vi "Panel.vi"(11 "MultiPlotPanel in":refnum<class "MultiPlotPanel.lvclass">) -> ()   [LabVIEW 2021, in "MultiStokePlot.lvlib" / "MultiPlotPanel.lvclass"]
uses:
  MultiPlotPanel.lvclass
  C:/Program Files/National Instruments/LabVIEW 2021/vi.lib/IlluminatedG/IG OOPanel/OOPanel/Panel/Panel.lvclass
  SubVIs/Window Position and plot number.ctl
  SubVIs/Window Position.ctl
  SubVIs/Loop Data.ctl
  <vilib>/IlluminatedG/IG OOPanel/OOPanel/Manager/Manager.lvclass
  SubVIs/Panel Map.ctl
  SubVIs/Panel Map Data.ctl
  <userlib>/bjustice/RocketPlot/Classes/RocketPlotPanel/RocketPlotPanel.lvclass
  <vilib>/IlluminatedG/IG OOPanel/OOPanel/Panel/Panel Events.ctl
  <vilib>/IlluminatedG/IG OOPanel/OOPanel/Panel/Visbility Event Data.ctl
  <vilib>/IlluminatedG/IG OOPanel/OOPanel/Visibility State.ctl
  <vilib>/IlluminatedG/IG OOPanel/OOPanel/Close Reason.ctl
  <vilib>/Utility/miscctls.llb/LVPointTypeDef.ctl
  <userlib>/bjustice/RocketPlot/Classes/RocketPlotHandle/SubVIs/callback data.ctl
  <userlib>/bjustice/RocketPlot/Classes/RocketPlotHandle/SubVIs/callback type.ctl
  MultiPlotPanel.lvclass/MultiPlotPanel.ctl
  <userlib>/bjustice/RocketPlot/Classes/RocketPlotHandle/SubVIs/callback maximize data.ctl
  <vilib>/IlluminatedG/IG OOPanel/OOPanel/Panel/Panel.lvclass
  <userlib>/bjustice/RocketPlot/Classes/RocketPlotHandle/RocketPlotHandle.lvclass
  <vilib>/IlluminatedG/IG OOPanel/OOPanel/OOPanel.lvlib
panel:
  in  "Selection":T1[](array[typedef]) {"Plot Bounds (%)"."Bottom (%)" format="%.2f"; "Plot Bounds (%)"."Top (%)" format="%.2f"; "Plot Bounds (%)"."Right (%)" format="%.2f"; "Plot Bounds (%)"."Left (%)" format="%.2f"}
  in  "Select Layout (spoof)":bool
  in  "Select Layout":bool
  in  "Save Layout (spoof)":bool
  in  "Save Layout":bool
  in  "Load Layout (spoof)":bool
  in  "Load Layout":bool
  in  "Time to Plot":dbl=1800.0 format="%<%H:%M:%S>t"
  in  "Apply Time to Plot":bool
  out "Filename":string
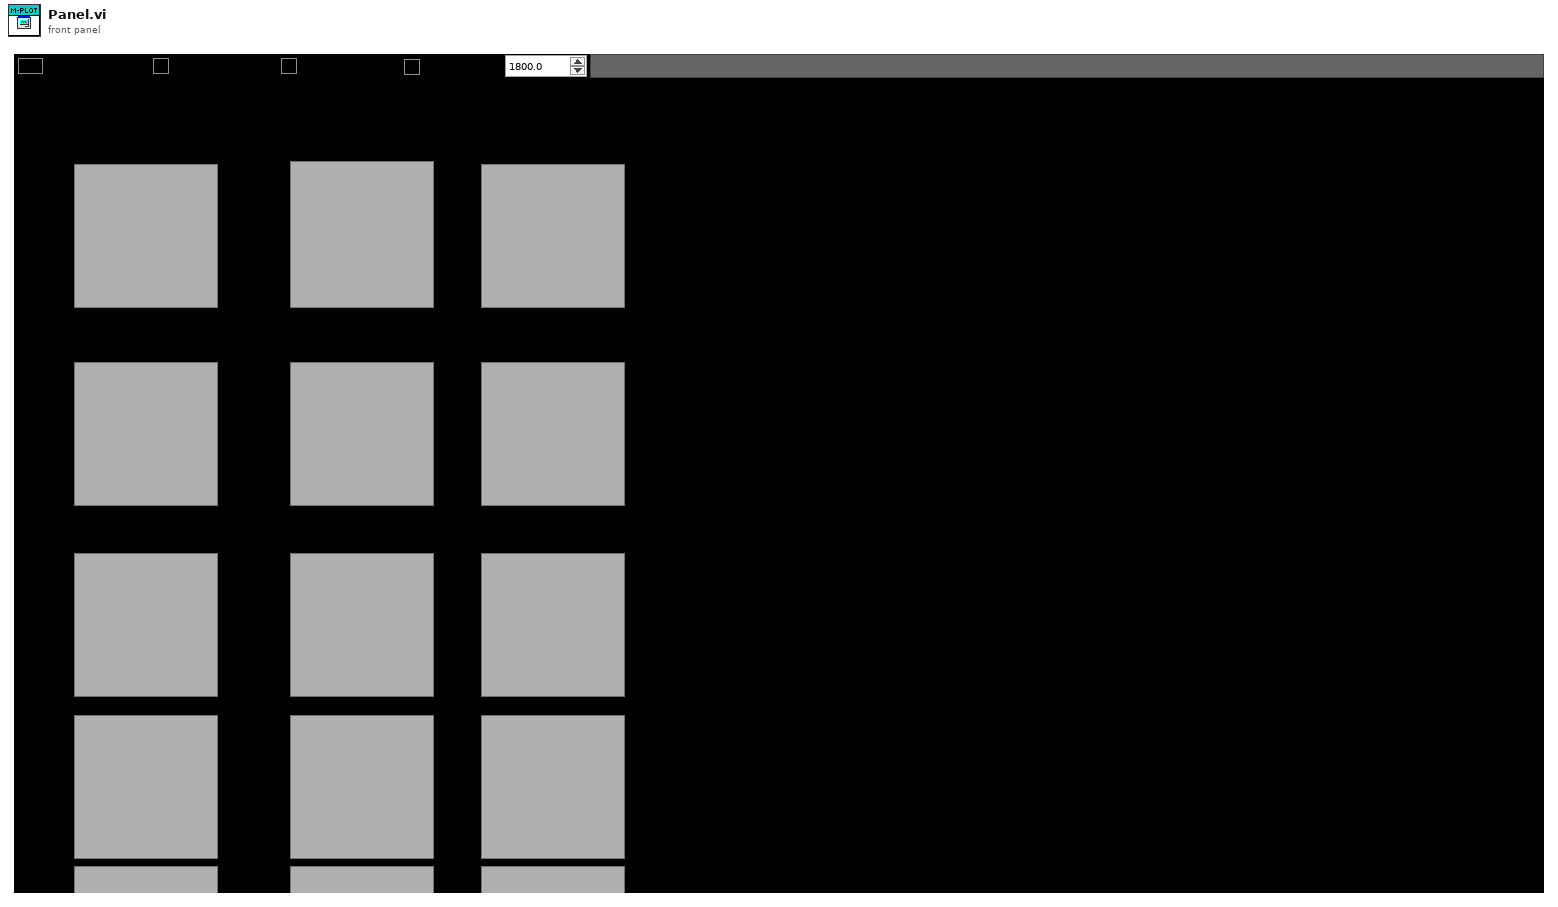
[diagram p1: front panel]
types:
  T1 = typedef "MultiStokePlot.lvlib/MultiPlotPanel.lvclass/Window Position and plot number.ctl" = cluster{"Plot Number":i32, "Plot Bounds (%)":T2}
  T2 = typedef "MultiStokePlot.lvlib/MultiPlotPanel.lvclass/Window Position.ctl" = cluster{"Left (%)":dbl, "Top (%)":dbl, "Right (%)":dbl, "Bottom (%)":dbl}
  T3 = typedef "LVPointTypeDef.ctl" = cluster{"Horizontal":i16, "Vertical":i16}
  T4 = typedef "MultiStokePlot.lvlib/MultiPlotPanel.lvclass/Loop Data.ctl" = cluster{"Panel Manager":refnum<class "Manager.lvclass">, "PanelMap":T5, "Fullscreen Plot Number":i32, "Panel Events":T7}
  T5 = typedef "MultiStokePlot.lvlib/MultiPlotPanel.lvclass/Panel Map.ctl" = map{i32, T6}
  T6 = typedef "MultiStokePlot.lvlib/MultiPlotPanel.lvclass/Panel Map Data.ctl" = cluster{"RocketPlotPanel":refnum<class "RocketPlotPanel.lvclass">, "Subpanel":refnum<vi>, "Plot Bounds (%)":T2, "max button":refnum<vi>}
  T7 = typedef "OOPanel.lvlib/Panel.lvclass/Panel Events.ctl" = cluster{"Visbility":refnum<user-event>, "Close":refnum<user-event>}
  T8 = typedef "RocketPlotHandle.lvclass/callback maximize data.ctl" = cluster{"Maximize?":bool, "max button":refnum<vi>}
  T9 = typedef "LVRectTypeDef.ctl" = cluster{"Left":i16, "Top":i16, "Right":i16, "Bottom":i16}
  T10 = typedef "OOPanel.lvlib/Visibility State.ctl" = enum16{"Idle", "Closed", "Hidden", "Visible", "Subpanel", "Hidden Subpanel"}
  T11 = typedef "RocketPlotHandle.lvclass/callback type.ctl" = enum16{"Maximize", "ShortcutMenu"}
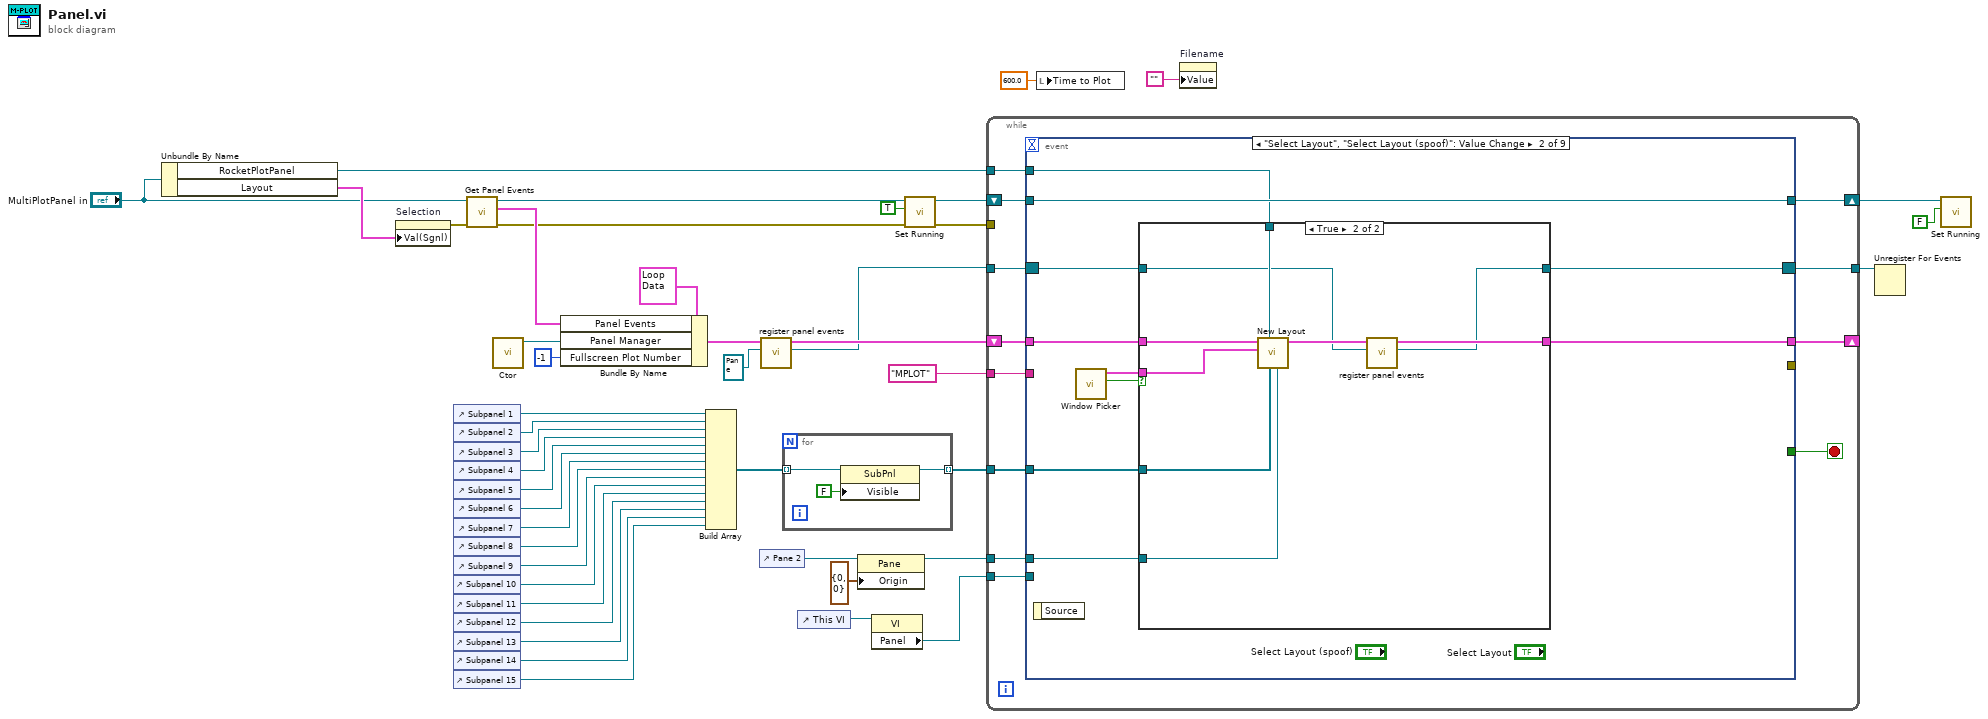
[diagram p0: block diagram]
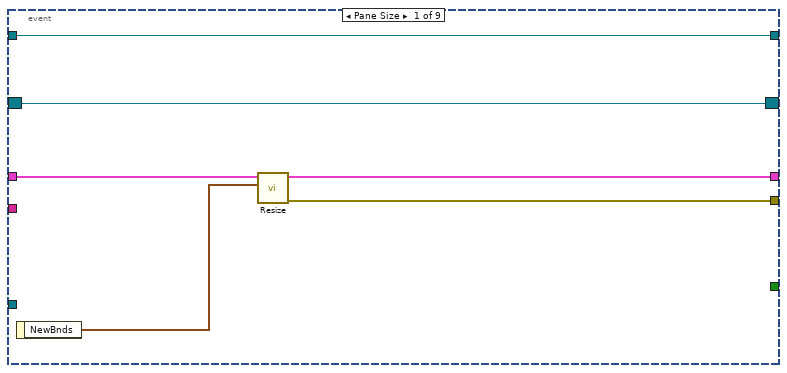
[diagram p2: hidden frame]
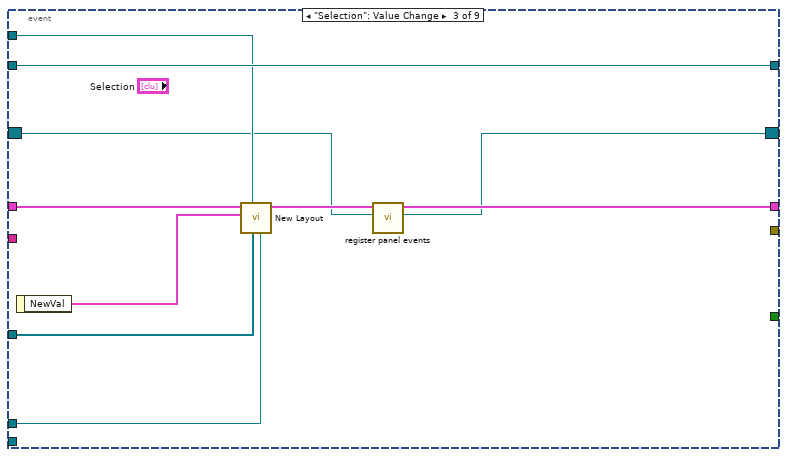
[diagram p4: hidden frame]
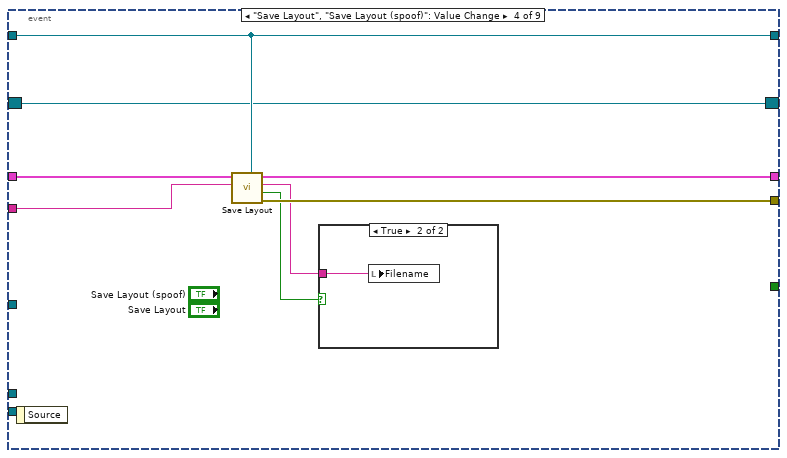
[diagram p5: hidden frame]
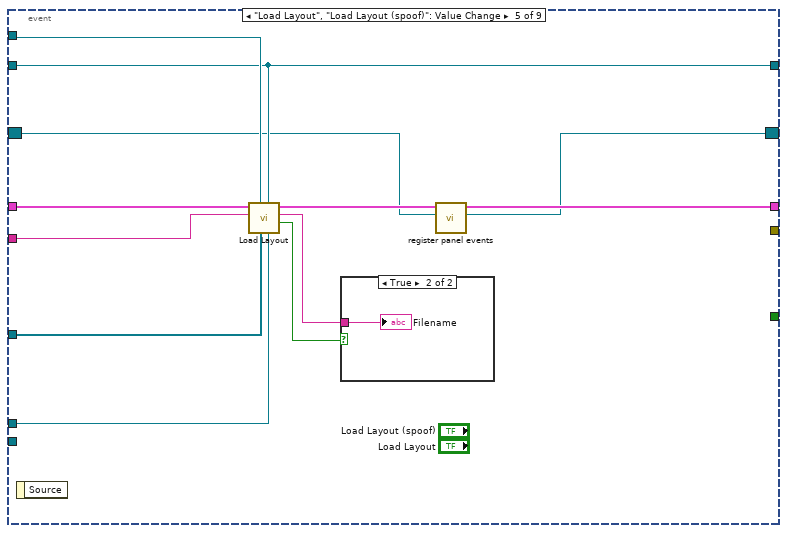
[diagram p7: hidden frame]
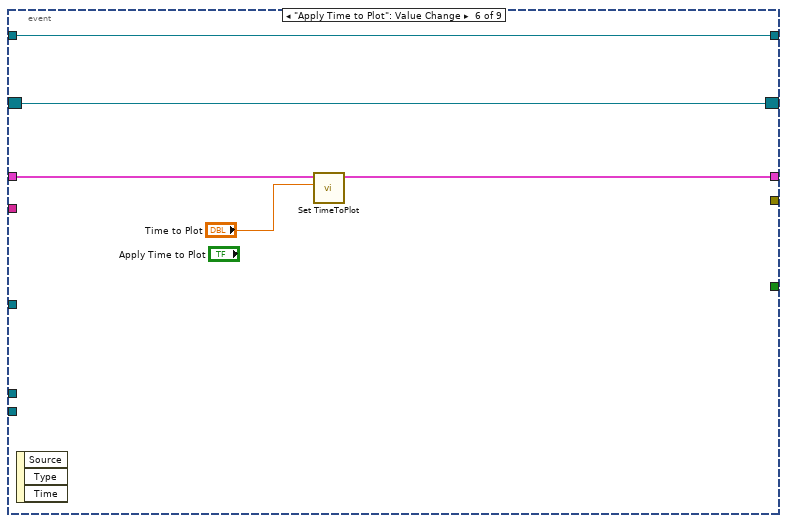
[diagram p9: hidden frame]
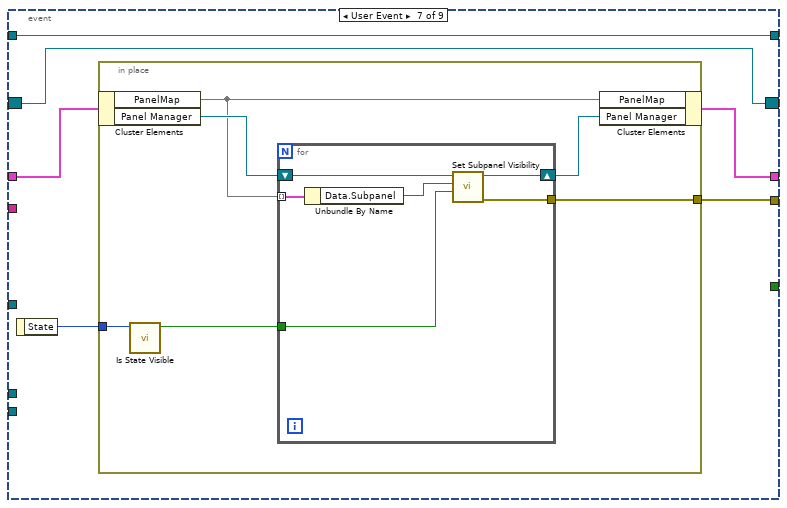
[diagram p10: hidden frame]
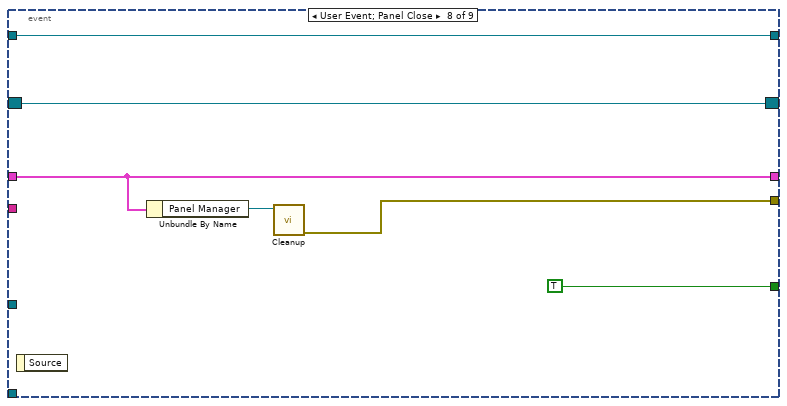
[diagram p11: hidden frame]
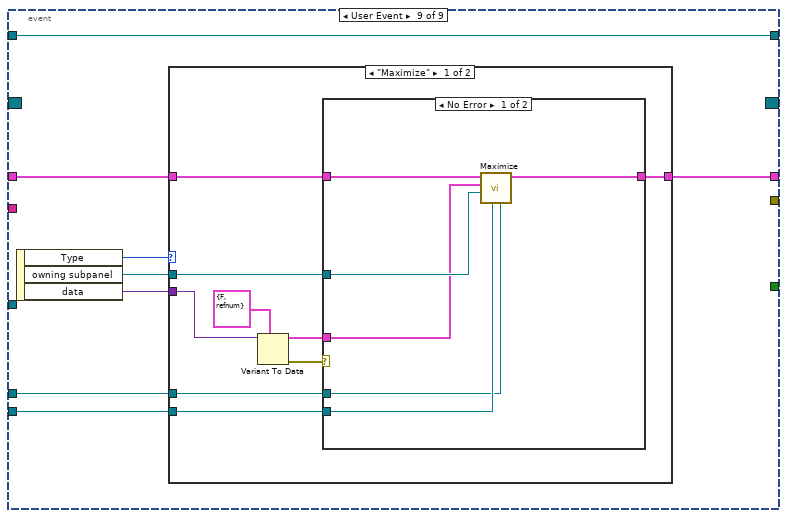
[diagram p12: hidden frame]
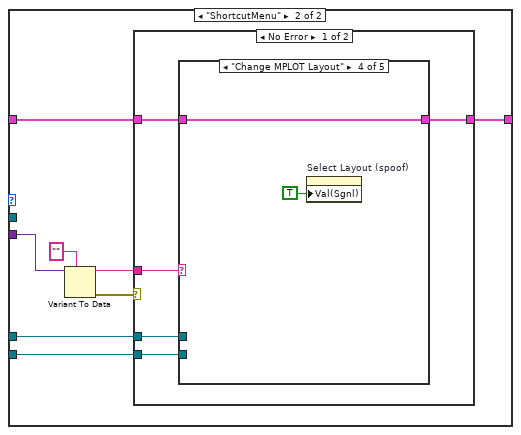
[diagram p14: hidden frame]
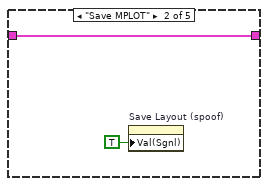
[diagram p16: hidden frame]
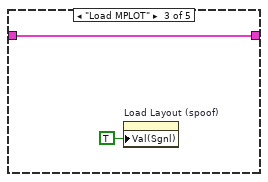
[diagram p17: hidden frame]
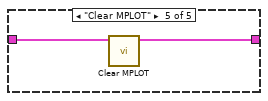
[diagram p18: hidden frame]
diagram:
  n1 = Unbundle By Name("MultiPlotPanel in") -> ("RocketPlotPanel"=w4:refnum<class "RocketPlotPanel.lvclass">, "Layout"=w20:T1[])
  n2 = property on="Selection" class="Arr (strict)"("Val(Sgnl)"=w20) -> (error out=w2:errorcluster)  [unwired: 2 in, 1 out]
  n3 = control-ref of="Subpanel 1"() -> (w43:refnum<vi>)
  n4 = control-ref of="Subpanel 2"() -> (w42:refnum<vi>)
  n5 = control-ref of="Subpanel 3"() -> (w41:refnum<vi>)
  n6 = control-ref of="Subpanel 4"() -> (w40:refnum<vi>)
  n7 = control-ref of="Subpanel 5"() -> (w39:refnum<vi>)
  n8 = control-ref of="Subpanel 6"() -> (w38:refnum<vi>)
  n9 = control-ref of="Subpanel 7"() -> (w37:refnum<vi>)
  n10 = control-ref of="Subpanel 8"() -> (w36:refnum<vi>)
  n11 = control-ref of="Subpanel 9"() -> (w35:refnum<vi>)
  n12 = control-ref of="Subpanel 10"() -> (w19:refnum<vi>)
  n13 = control-ref of="Subpanel 11"() -> (w18:refnum<vi>)
  n14 = control-ref of="Subpanel 12"() -> (w17:refnum<vi>)
  n15 = control-ref of="Subpanel 13"() -> (w16:refnum<vi>)
  n16 = control-ref of="Subpanel 14"() -> (w15:refnum<vi>)
  n17 = control-ref of="Subpanel 15"() -> (w14:refnum<vi>)
  n18 = call <vilib>:"Get Panel Events.vi"("error in (no error)"=w2, "Panel in"="MultiPlotPanel in") -> ("error out"=w5:errorcluster, "Panel Events"=w9:T7, "Panel out"=w24:refnum<class "MultiPlotPanel.lvclass">)  [unwired: 7 in]
  n19 = call <vilib>:"Ctor.vi"() -> ("Manager out"=w33:refnum<class "Manager.lvclass">)  [unwired: 10 in, 1 out]
  n20 = Bundle By Name(cluster=T4 {"Panel Manager"=refnum, "PanelMap"={}, "Fullscreen Plot Number"=0, "Panel Events"={"Visbility"=refnum, "Close"=refnum}} ("Cluster"), "Panel Events"=w9, "Panel Manager"=w33, "Fullscreen Plot Number"=-1) -> (w8:T4)
  n21 = Build Array(w43, w42, w41, w40, w39, w38, w37, w36, w35, w19, w18, w17, w16, w15, w14) -> (w29:refnum<vi>[])
  n22 = control-ref of="Pane 2"() -> (w32:refnum<vi>)
  n23 = call "register panel events.vi"("Event Registration Refnum"=refnum<event-registration> refnum, "Loop data in"=w8) -> ("Event Registration Refnum"=w6:refnum<event-registration>, "Loop data out"=w7:T4)  [unwired: 7 in, 1 out]
  n24 = for {
    tunnel: w29 -> [w48] mode=indexing
    tunnel: [w46] -> w28 mode=indexing
    n25 = property class="SubPnl"(reference=w48, "Visible"=FALSE) -> (reference out=w46:refnum<vi>)  [unwired: 1 in, 1 out]
  }
  n26 = control-ref of="This VI"() -> (w11:refnum<vi>)
  n27 = property class="Pane"(reference=w32, "Origin"=T3 {"Horizontal"=0, "Vertical"=0}) -> (reference out=w31:refnum<vi>)  [unwired: 1 in, 1 out]
  n28 = property class="VI"(reference=w11) -> ("Panel"=w10:refnum<vi>)  [unwired: 1 in, 2 out]
  n29 = call <vilib>:"Set Running.vi"("error in (no error)"=w5, "Running"=TRUE, "Panel in"=w24) -> ("error out"=w21:errorcluster, "Panel out"=w23:refnum<class "MultiPlotPanel.lvclass">)  [unwired: 7 in]
  n30 = while {
    shift-right: [w56] -> _
    shift-left: w7 -> [w57]
    tunnel: w28 -> [w55]
    tunnel: w31 -> [w54]
    tunnel: w6 -> [w49]
    tunnel: [w53] -> w27
    tunnel: "MPLOT" -> [w52]
    shift-right: [w58] -> w45
    shift-left: w23 -> [w59]
    tunnel: w4 -> [w51]
    tunnel: w21 -> [_]
    tunnel: w10 -> [w50]
    stop <- w60 stop-if-true
    n31 = event shown="[1] \"Select Layout\", \"Select Layout (spoof)\": Value Change" {
      selector: w49 -> [w61 w67 w88 w98 w107 w120 w125 w143 _]
      dyn-events: [w61 w68 w89 w98 w108 w120 w125 w143 _] -> w53
      timeout: _ -> [_ _ _ _ _ _ _ _ _]
      tunnel: [_ _ _ _ _ _ _ TRUE _] -> w60
      tunnel: w59 -> [w63 w72 w96 w99 w111 w121 w128 w147 w156]
      tunnel: [w63 w72 w96 w99 w111 w121 w128 w147 w156] -> w58
      tunnel: w57 -> [w66 w74 w97 w105 w118 w124 w130 w145 w151]
      tunnel: [w64 w73 w90 w104 w109 w123 w127 w145 w150] -> w56
      tunnel: w55 -> [_ w71 w95 _ w116 _ _ _ _]
      tunnel: w54 -> [_ w70 w94 _ w115 _ _ _ w149]
      tunnel: w52 -> [_ _ _ w103 w117 _ _ _ _]
      tunnel: [w62 _ _ w102 _ _ w126 w144 _] -> _
      tunnel: w51 -> [_ w69 w93 _ w112 _ _ _ _]
      tunnel: w50 -> [_ _ _ _ _ _ _ _ w152]
      event Pane Size {
        n32 = event-data() -> ("NewBnds"=w65:T9)  [unwired: 1 in]
        n33 = call "Resize.vi"("Pane.Content Area Rect"=w65, "Loop data in"=w66) -> ("error out"=w62:errorcluster, "Loop data out"=w64:T4)  [unwired: 8 in]
      }
      event "Select Layout", "Select Layout (spoof)": Value Change {
        n34 = event-data() -> ()  [unwired: 1 in, 1 out]
        n35 = call "Window Picker.vi"() -> ("Selected?"=w76:bool, "Selection"=w75:T1[])  [unwired: 10 in]
        n36 = case shown="True" w76 {
          tunnel: w75 -> [_ w85]
          tunnel: w74 -> [w78 w87]
          tunnel: [w78 w81] -> w73
          tunnel: w69 -> [_ w86]
          tunnel: w71 -> [_ w84]
          tunnel: w70 -> [_ w83]
          tunnel: [w77 w80] -> w68
          tunnel: w67 -> [w77 w79]
          frame False {
          }
          frame True {
            n37 = call "New Layout.vi"("PlotPane"=w83, "Subpanel Refs (ALL)"=w84, "RocketPlotPanel Type"=w86, "Layout"=w85, "Loop data in"=w87) -> ("Loop data out"=w82:T4)  [unwired: 5 in, 1 out]
            n38 = call "register panel events.vi"("Event Registration Refnum"=w79, "Loop data in"=w82) -> ("Event Registration Refnum"=w80:refnum<event-registration>, "Loop data out"=w81:T4)  [unwired: 7 in, 1 out]
          }
        }
      }
      event "Selection": Value Change {
        n39 = event-data() -> ("NewVal"=w92:T1[])  [unwired: 1 in]
        n40 = call "New Layout.vi"("PlotPane"=w94, "Subpanel Refs (ALL)"=w95, "RocketPlotPanel Type"=w93, "Layout"=w92, "Loop data in"=w97) -> ("Loop data out"=w91:T4)  [unwired: 5 in, 1 out]
        n41 = call "register panel events.vi"("Event Registration Refnum"=w88, "Loop data in"=w91) -> ("Event Registration Refnum"=w89:refnum<event-registration>, "Loop data out"=w90:T4)  [unwired: 7 in, 1 out]
      }
      event "Save Layout", "Save Layout (spoof)": Value Change {
        n42 = event-data() -> ()  [unwired: 1 in, 1 out]
        n43 = call "Save Layout.vi"("MultiPlotPanel in"=w99, "file extension"=w103, "Loop data in"=w105) -> ("error out"=w102:errorcluster, "Valid save?"=w101:bool, "Filename"=w100:string, "Loop data out"=w104:T4)  [unwired: 5 in]
        n44 = case shown="True" w101 {
          tunnel: w100 -> [_ w106]
          frame False {
          }
          frame True {
            n45 = local write "Filename"(w106) -> ()
          }
        }
      }
      event "Load Layout", "Load Layout (spoof)": Value Change {
        n46 = event-data() -> ()  [unwired: 1 in, 1 out]
        n47 = call "Load Layout.vi"("PlotPane"=w115, "MultiPlotPanel in"=w111, "Subpanel Refs (ALL)"=w116, "RocketPlotPanel Type"=w112, "file extension"=w117, "Loop data in"=w118) -> ("Valid load?"=w114:bool, "Filename"=w113:string, "Loop data out"=w110:T4)  [unwired: 2 in, 1 out]
        n48 = case shown="True" w114 {
          tunnel: w113 -> [_ w119]
          frame False {
          }
          frame True {
            "Filename" <- w119
          }
        }
        n49 = call "register panel events.vi"("Event Registration Refnum"=w107, "Loop data in"=w110) -> ("Event Registration Refnum"=w108:refnum<event-registration>, "Loop data out"=w109:T4)  [unwired: 7 in, 1 out]
      }
      event "Apply Time to Plot": Value Change {
        n50 = event-data() -> ()  [unwired: 1 in, 3 out]
        n51 = call "Set TimeToPlot.vi"("Time to Plot"="Time to Plot", "Loop data in"=w124) -> ("Loop data out"=w123:T4)  [unwired: 8 in, 1 out]
      }
      event User Event {
        n52 = event-data() -> ("State"=w129:T10)  [unwired: 1 in]
        n53 = in-place {
          in-place-border: w129 -> [w134]
          in-place-border: [w132] -> w126
          n54 = in-place-cluster #1(w130) -> ("PanelMap"=w131:T5, "Panel Manager"=w136:refnum<class "Manager.lvclass">)
          n55 = call <vilib>:"Is State Visible.vi"("Visibility"=w134) -> ("Visible"=w133:bool)  [unwired: 10 in]
          n56 = for {
            shift-right: [w141] -> w135
            shift-left: w136 -> [w142]
            tunnel: w133 -> [w140]
            tunnel: [w139] -> w132
            tunnel: w131 -> [w138] mode=indexing
            n57 = Unbundle By Name(w138) -> ("Data.Subpanel"=w137:refnum<vi>)
            n58 = call <vilib>:"Set Subpanel Visibility.vi"("Visible"=w140, "SubPanel"=w137, "Manager in"=w142) -> ("error out"=w139:errorcluster, "Manager out"=w141:refnum<class "Manager.lvclass">)  [unwired: 7 in]
          }
          n59 = in-place-cluster #1("PanelMap"=w131, "Panel Manager"=w135) -> (w127:T4)
        }
      }
      event User Event; Panel Close {
        n60 = event-data() -> ()  [unwired: 1 in, 1 out]
        n61 = Unbundle By Name(w145) -> ("Panel Manager"=w146:refnum<class "Manager.lvclass">)
        n62 = call <vilib>:"Cleanup.vi"("Manager in"=w146) -> ("error out"=w144:errorcluster)  [unwired: 8 in, 2 out]
      }
      event User Event {
        n63 = event-data() -> ("Type"=w155:T11, "owning subpanel"=w154:refnum<vi>, "data"=w153:variant)  [unwired: 1 in]
        n64 = case shown="\"Maximize\"" w155 {
          tunnel: w151 -> [w165 w180]
          tunnel: [w164 w179] -> w150
          tunnel: w154 -> [w163 _]
          tunnel: w149 -> [w157 w178]
          tunnel: w152 -> [w162 w177]
          tunnel: w153 -> [w161 w175]
          frame "Maximize" {
            n65 = Variant To Data(type=T8 {"Maximize?"=FALSE, "max button"=refnum} ("Cluster"), Variant=w161) -> (data=w160:T8, error out=w159:errorcluster)  [unwired: 1 in]
            n66 = case shown="No Error" w159 {
              tunnel: w165 -> [w171 w172]
              tunnel: [w170 w172] -> w164
              tunnel: w163 -> [w169 _]
              tunnel: w162 -> [w168 _]
              tunnel: w157 -> [w167 _]
              tunnel: w160 -> [w166 _]
              frame No Error {
                n67 = call "Maximize.vi"("PlotPane"=w167, "Front Panel"=w168, "owning subpanel"=w169, "maximize button data"=w166, "Loop data in"=w171) -> ("Loop data out"=w170:T4)  [unwired: 5 in, 1 out]
              }
              frame Error {
              }
            }
          }
          frame "ShortcutMenu" {
            n68 = Variant To Data(type="", Variant=w175) -> (data=w174:string, error out=w173:errorcluster)  [unwired: 1 in]
            n69 = case shown="No Error" w173 {
              tunnel: w180 -> [w185 w195]
              tunnel: [w184 w195] -> w179
              tunnel: w178 -> [w183 _]
              tunnel: w177 -> [w182 _]
              tunnel: w174 -> [w181 _]
              frame No Error {
                n70 = case shown="\"Change MPLOT Layout\"" w181 {
                  tunnel: w185 -> [w186 w187 w189 w191 w194]
                  tunnel: [w186 w187 w189 w191 w193] -> w184
                  tunnel: w183 -> [_ _ _ _ _]
                  tunnel: w182 -> [_ _ _ _ _]
                  frame Default {
                  }
                  frame "Save MPLOT" {
                    n71 = property on="Save Layout (spoof)" class="Bool (strict)"("Val(Sgnl)"=TRUE ("Value (Signaling)")) -> ()  [unwired: 2 in, 2 out]
                  }
                  frame "Load MPLOT" {
                    n72 = property on="Load Layout (spoof)" class="Bool (strict)"("Val(Sgnl)"=TRUE ("Value (Signaling)")) -> ()  [unwired: 2 in, 2 out]
                  }
                  frame "Change MPLOT Layout" {
                    n73 = property on="Select Layout (spoof)" class="Bool (strict)"("Val(Sgnl)"=TRUE ("Value (Signaling)")) -> ()  [unwired: 2 in, 2 out]
                  }
                  frame "Clear MPLOT" {
                    n74 = call "Clear MPLOT.vi"("loop data in"=w194) -> ("loop data out"=w193:T4)  [unwired: 10 in]
                  }
                }
              }
              frame Error {
              }
            }
          }
        }
      }
    }
  }
  n75 = local write "Time to Plot"(600.0 ("Time to Plot")) -> ()
  n76 = property on="Filename" class="Str"("Value"="") -> ()  [unwired: 2 in, 2 out]
  n77 = Unregister For Events(event registration refnum=w27) -> ()  [unwired: 1 in, 1 out]
  n78 = call <vilib>:"Set Running.vi"("Running"=FALSE, "Panel in"=w45) -> ()  [unwired: 8 in, 2 out]
